vi "2100_Scan USID.vi"(5 "Published Data Id":string="Num_Of_USID", 7 "Potential_USID_Array":T4[](array[typedef])=[1, 2, 4, 7, 8, 9, 13, 15] max=15, 8 "Error In":errorcluster, 9 "Reg_Address_to_Read":T2={"First Reg Address"=31, "Num of Reg to Read"=1} {"Num of Reg to Read" min=1; "First Reg Address" format="%.0x"}, 10 "Pins":string[](array[string])=["CLK", "SDA"], 11 "Semiconductor Module Context":T1) -> (0 "Error Out":errorcluster, 2 "DUT_USID":u8, 3 "USIDs_Detected":u8[](array[numeric]))   [LabVIEW 2013]
uses:
  Controls/USID.ctl
  <vilib>/NI_TestStand_SemiconductorModule/NI_TestStand_Semiconductor_Module.lvlibp/PinMap/General/SemiconductorModuleContext.ctl
  Controls/Reg_Address_Data.ctl
  <vilib>/NI_TestStand_SemiconductorModule/NI_TestStand_Semiconductor_Module.lvlibp/PinMap/General/Publish/PublishDataDoubleFunctionalTest.vi
  <vilib>/NI_TestStand_SemiconductorModule/NI_TestStand_Semiconductor_Module.lvlibp
panel:
  out "Converted Data":T3 {"Register" max=31 format="%.0x"; "Slave Address" max=15 format="%.0x"}
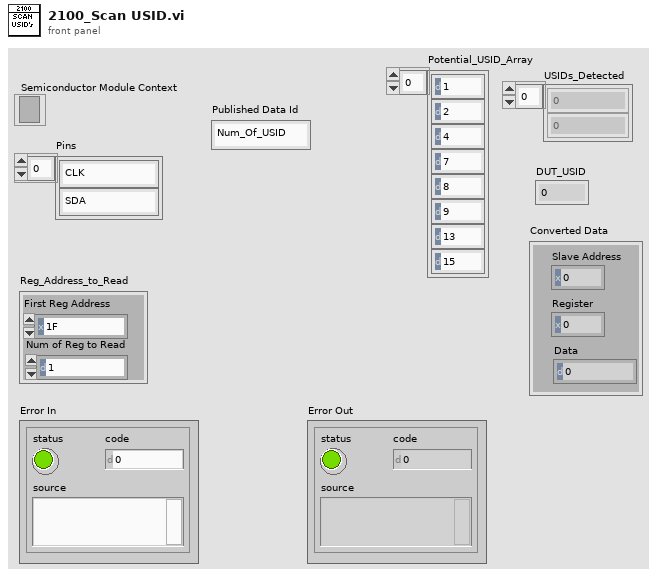
[diagram p1: front panel]
types:
  T1 = typedef "NI_TestStand_Semiconductor_Module.lvlibp/SemiconductorModuleContext.ctl" = refnum<k7>
  T2 = cluster{"First Reg Address":u8, "Num of Reg to Read":u8}
  T3 = cluster{"Slave Address":u8, "Register":u8, "Data":u8}
  T4 = typedef "USID.ctl" = u8
  T5 = typedef "Reg_Address_Data.ctl" = cluster{"Address":u8, "Data":u8}
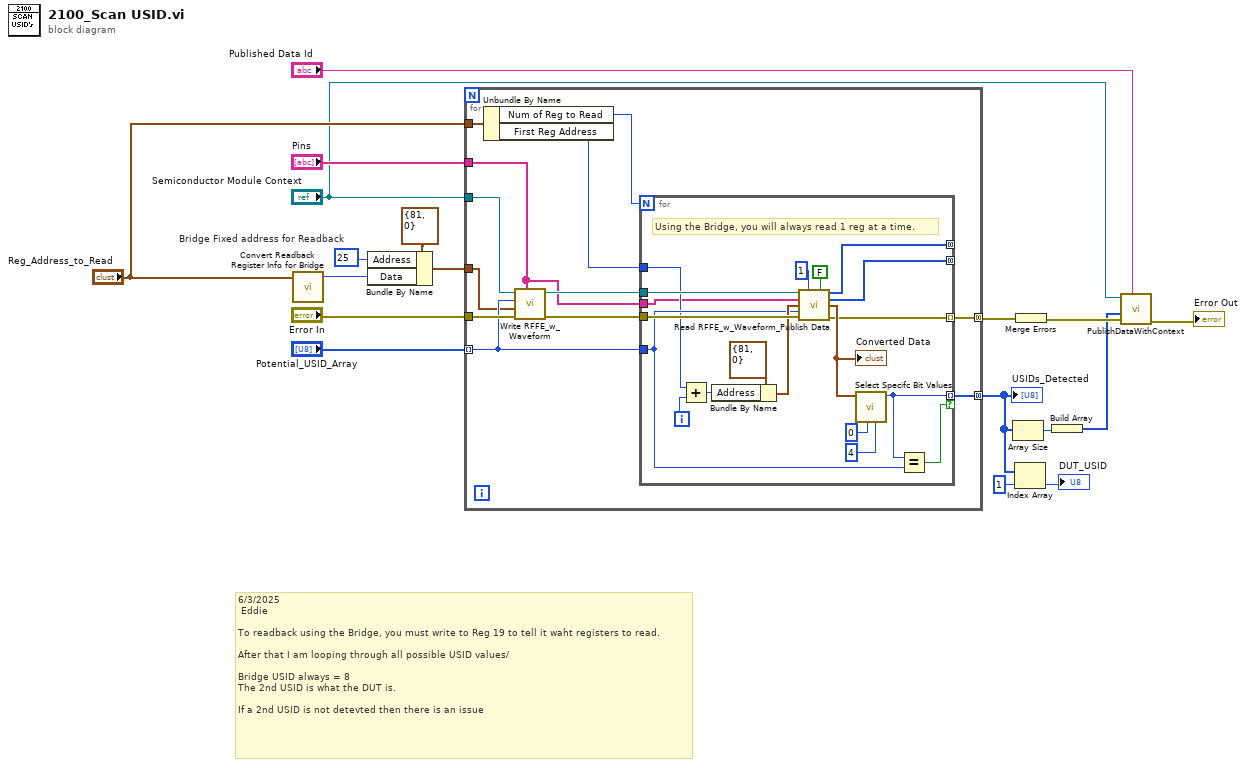
[diagram p0: block diagram]
diagram:
  w15 = u8 25  # Bridge Fixed address for Readback
  # "6/3/2025\n Eddie\n\nTo readback using the Bridge, you must write to Reg 19 to tell it waht registers to read.\n\nAfter that I am looping through all possible USID values/ \n\nBridge USID always = 8\nThe 2nd USID is what the DUT is.\n\nIf a 2nd USID is not detevted then there is an issue"
  n1 = call "Convert Readback Register Info for Bridge.vi"("Reg_Address_to_Read"="Reg_Address_to_Read") -> ("number"=w16:u32)  [unwired: 4 in]
  n2 = Bundle By Name(cluster=T5 {"Address"=81, "Data"=0} ("Reg_Address_Data"), "Address"=w15, "Data"=w16) -> (w13:T5)
  n3 = for {
    tunnel: "Potential_USID_Array" -> [w24] mode=indexing
    tunnel: [w29] -> w3 mode=concatenating
    tunnel: "Semiconductor Module Context" -> [w28]
    tunnel: "Error In" -> [w25]
    tunnel: w13 -> [w23]
    tunnel: "Reg_Address_to_Read" -> [w22]
    tunnel: "Pins" -> [w20]
    tunnel: [w19] -> w7 mode=concatenating
    n4 = Unbundle By Name(w22) -> ("Num of Reg to Read"=w21:u8, "First Reg Address"=w30:u8)
    n5 = call "Write RFFE_w_Waveform.vi"("Pins"=w20, "error in (no error)"=w25, "Reg_Address_Data"=w23, "USID"=w24, "Semiconductor Module Context"=w28) -> ("error out"=w26:errorcluster, "Semiconductor Module Context Out"=w27:T1)  [unwired: 5 in]
    n6 = for {
      N: w21 -> [_]
      tunnel: w24 -> [w34]
      tunnel: w30 -> [w33]
      tunnel: [w44] -> w29 mode=indexing if=w43
      tunnel: [w41] -> _ mode=concatenating
      tunnel: [w40] -> _ mode=concatenating
      tunnel: w27 -> [w37]
      tunnel: w26 -> [w36]
      tunnel: w20 -> [w32]
      tunnel: [w31] -> w19 mode=indexing
      i -> [w47]
      # "Using the Bridge, you will always read 1 reg at a time."
      n7 = Add(x=w33, y=w47) -> (x+y=w46:i32)
      n8 = Bundle By Name(cluster=T5 {"Address"=81, "Data"=0} ("Reg_Address_Data"), "Address"=w46) -> (w35:T5)
      n9 = call "Read RFFE_w_Waveform_Publish Data.vi"("Semiconductor Module Context"=w37, "Num_Reg_to_Read"=u8 1, "Publish_Data?"=FALSE, "Pins"=w32, "Reg_Address_Data"=w35, "USID"=w34, "Error In"=w36) -> ("Ext_Read_Reg"=w41:i32[], "Ext_Read_Data"=w40:u8[], "Converted Data"=w39:T3, "Error Out"=w31:errorcluster)  [unwired: 4 in, 1 out]
      "Converted Data" <- w39
      n10 = call "Select Specifc Bit Values.vi"("#ofBits"=u8 4, "Bit_Location(LSB)"=u8 0, "Converted Data"=w39) -> ("Bits"=w44:u8)  [unwired: 8 in]
      n11 = Equal?(x=w44, y=w34) -> (x = y?=w43:bool)
    }
  }
  "USIDs_Detected" <- w3
  n12 = Array Size(array=w3) -> (size(s)=w9:i32)
  n13 = Index Array(array=w3, index=1) -> (element=→"DUT_USID":u8)
  n14 = Merge Errors(w7) -> (w10:errorcluster)
  n15 = Build Array(w9) -> (w8:i32[])
  n16 = call-poly <vilib>:"PublishDataWithContext.vi"("Published Data Id"="Published Data Id", "error in (no error)"=w10, "Data In"=w8, "Semiconductor Module Context"="Semiconductor Module Context") -> ("error out"=→"Error Out":errorcluster)  [unwired: 6 in, 1 out]
